vi "DigitalOutCounterSet.vi"(4 "counter":u32, 6 "initlevel":i32, 7 "ch":i32, 8 "error in (no error)":errorcluster caption="错误输入（无错误）", 9 "counter_l":u32=1, 10 "counter_h":u32=1, 11 "handle":u64) -> (0 "error out":errorcluster caption="错误输出", 2 "function return":i32, 3 "handle out":u64)   [LabVIEW 2018]
doc: "Set pos. or neg. Supply voltage"
uses:
  InstrumentsPlayground.lvlib
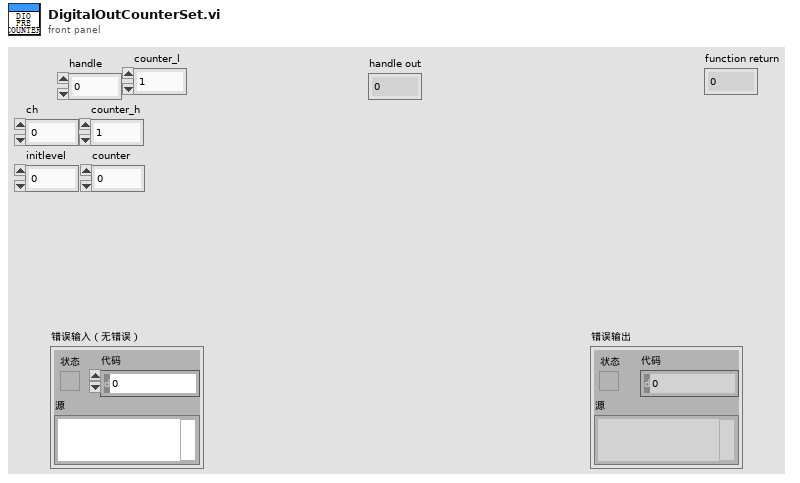
[diagram p1: front panel]
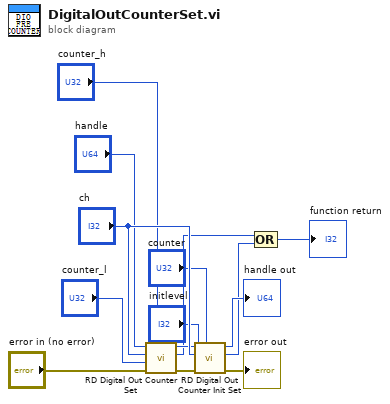
[diagram p0: block diagram]
diagram:
  n1 = call "RD Digital Out Counter Set.vi"("counter_h"="counter_h", "error in (no error)"="error in (no error)", "counter_l"="counter_l", "ch"="ch", "handle"="handle") -> ("error out"=w10:errorcluster, "function return"=w3:i32, "handle out"=w8:u64)  [unwired: 4 in]
  n2 = call "RD Digital Out Counter Init Set.vi"("counter"="counter", "error in (no error)"=w10, "initlevel"="initlevel", "ch"="ch", "handle"=w8) -> ("error out"=→"error out":errorcluster, "function return"=w6:i32, "handle out"=→"handle out":u64)  [unwired: 4 in]
  n3 = Compound Arithmetic op=OR ("复合运算")(w3, w6) -> (→"function return":i32)
